vi "addComponent.vi"(0 "HGF_Composite":refnum<class "HGF_Composite.lvclass">, 2 "HGF_Component":refnum<class "HGF_Component.lvclass">, 5 "error in (no error)":errorcluster) -> (14 "dup HGF_Composite":refnum<class "HGF_Composite.lvclass">, 19 "error out":errorcluster)   [LabVIEW 2014, in "HGF_BaseClasses.lvlib" / "HGF_Composite.lvclass"]
doc: "Add Component object to Composite object."
uses:
  HGF_Composite.lvclass
  HGF_Component/HGF_Component.lvclass
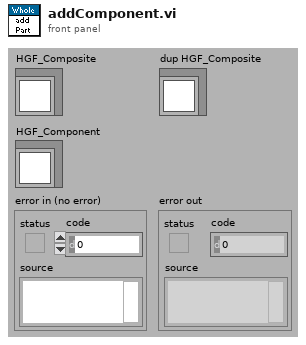
[diagram p1: front panel]
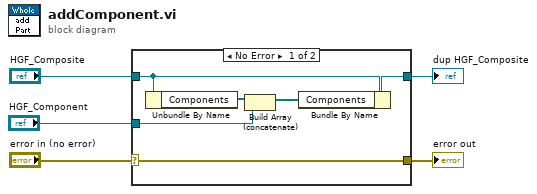
[diagram p0: block diagram]
diagram:
  n1 = case shown="No Error" "error in (no error)" {
    selector: "error in (no error)" -> [w11 w13]
    tunnel: [w11 w13] -> w4
    tunnel: [w6 w12] -> w2
    tunnel: "HGF_Composite" -> [w7 w12]
    tunnel: "HGF_Component" -> [w9 _]
    frame No Error {
      n2 = Unbundle By Name(w7) -> ("Components"=w10:refnum<class "HGF_Component.lvclass">[])
      n3 = Build Array (concatenate)(w10, w9) -> (w8:refnum<class "HGF_Component.lvclass">[])
      n4 = Bundle By Name(cluster=w7, "Components"=w8) -> (w6:refnum<class "HGF_Composite.lvclass">)
    }
    frame Error {
    }
  }
  "error out" <- w4
  "dup HGF_Composite" <- w2
